vi "Move Lift For Inches.vi"(10 "Distance Back Up":dbl=6.0 format="%#_13g", 11 "Distance Down":dbl=6.0 format="%#_13g") -> ()   [LabVIEW 2014]
uses:
  Global Variables.vi
panel:
  out "Done":bool
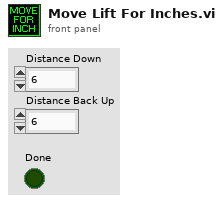
[diagram p1: front panel]
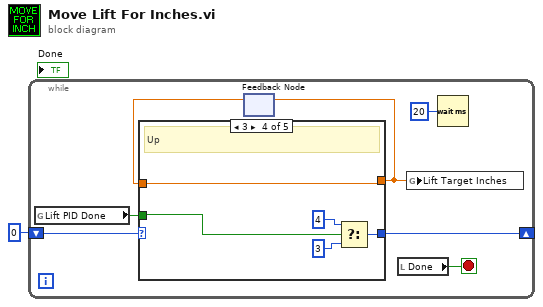
[diagram p0: block diagram]
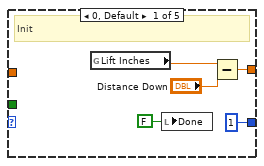
[diagram p2: hidden frame]
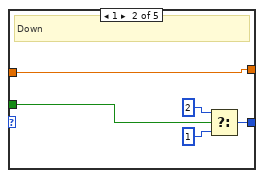
[diagram p3: hidden frame]
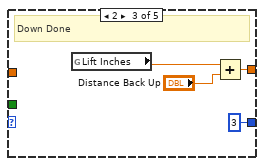
[diagram p4: hidden frame]
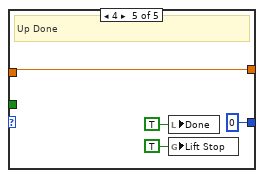
[diagram p5: hidden frame]
diagram:
  n1 = while {
    shift-right: [w6] -> _
    shift-left: 0 ("f") -> [w7]
    stop <- w2 stop-if-true
    n2 = global read "Global Variables.vi" "Lift PID Done"() -> (w4:bool)
    n3 = feedback #1() -> (w5:dbl)  [unwired: 1 in]
    n4 = case shown="3" w7 {
      tunnel: [w13 w18 w20 w27 w29] -> w3
      tunnel: [1 ("f") w17 3 ("f") w25 0 ("f")] -> w6
      tunnel: w5 -> [_ w18 _ w27 w29]
      tunnel: w4 -> [_ w16 _ w23 _]
      frame 0, Default {
        # "Init"
        n5 = global read "Global Variables.vi" "Lift Inches"() -> (w12:dbl)
        n6 = local write "Done"(FALSE ("Done")) -> ()
        n7 = Subtract(x=w12, y="Distance Down") -> (x-y=w13:dbl)
      }
      frame 1 {
        # "Down"
        n8 = Select(t=2 ("f"), s=w16, f=1) -> (s? t:f=w17:i32)
      }
      frame 2 {
        # "Down Done"
        n9 = global read "Global Variables.vi" "Lift Inches"() -> (w22:dbl)
        n10 = Add(x=w22, y="Distance Back Up") -> (x+y=w20:dbl)
      }
      frame 3 {
        # "Up"
        n11 = Select(t=4 ("f"), s=w23, f=3) -> (s? t:f=w25:i32)
      }
      frame 4 {
        # "Up Done"
        n12 = local write "Done"(TRUE ("Done")) -> ()
        n13 = global write "Global Variables.vi" "Lift Stop"(TRUE ("Lift Stop")) -> ()
      }
    }
    n14 = feedback-in #1(w3) -> ()
    n15 = local read "Done"() -> (w2:bool)
    n16 = global write "Global Variables.vi" "Lift Target Inches"(w3) -> ()
    n17 = Wait (ms)(milliseconds to wait=u32 20) -> ()  [unwired: 1 out]
  }
